vi "Pre Launch Init.vi"(11 "Nested in":refnum<class "test.lvclass">) -> (0 "error out":errorcluster, 3 "Nested out":refnum<class "test.lvclass">)   [LabVIEW 2020, in "test.lvlib" / "test.lvclass"]
doc: "(<B>Filename</B>: Actor Framework.lvlib:Actor.lvclass:Pre Launch Init.vi)\n\nDefines behavior that occurs after the Launch Nested Actor method is invoked but before the actor's Actor Core method begins running.\n\nBy default, this method does nothing. A descendant class may override it to define behavior."
uses:
  test.lvclass
  classes/vna-drivers/liteVNA/VD-settings_status.ctl
  test.lvclass/test.ctl
  <vilib>/ActorFramework/Actor/Actor.lvclass
  classes/vna-drivers/liteVNA/VD-LV-LiteVNA.lvclass
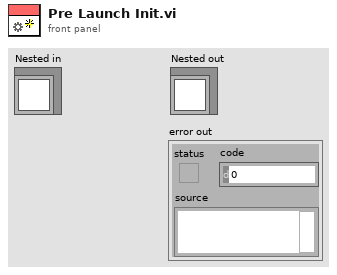
[diagram p1: front panel]
types:
  T1 = typedef "VD-LV-LiteVNA.lvclass/VD-settings_status.ctl" = cluster{"Start [Hz]":u64, "Span [Hz]":u64, "Stop [Mhz]":u64, "Number of points #":u16, "Sample Average #":u16}
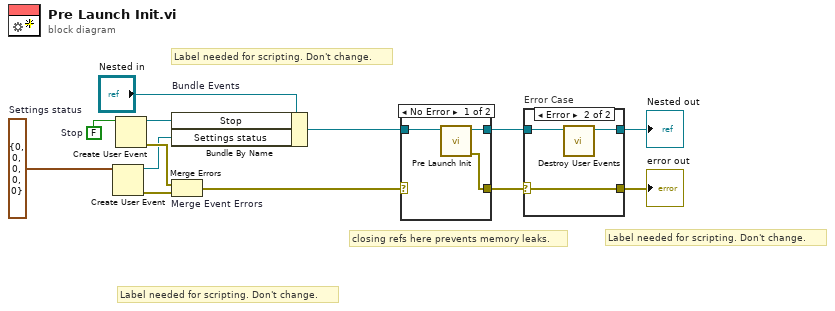
[diagram p0: block diagram]
diagram:
  w3 = T1 {"Start [Hz]"=0, "Span [Hz]"=0, "Stop [Mhz]"=0, "Number of points #"=0, "Sample Average #"=0}  # Settings status
  w12 = FALSE  # Stop
  # "Label needed for scripting. Don't change."
  # "Label needed for scripting. Don't change."
  # "Label needed for scripting. Don't change."
  # "closing refs here prevents memory leaks."
  n1 = Create User Event(user event datatype=w3) -> (user event=w2:refnum<user-event>, error out=w1:errorcluster)  [unwired: 1 in]
  n2 = Create User Event(user event datatype=w12) -> (user event=w9:refnum<user-event>, error out=w11:errorcluster)  [unwired: 1 in]
  n3 = Bundle By Name "Bundle Events"(cluster="Nested in", "Stop"=w9, "Settings status"=w2) -> (w6:refnum<class "test.lvclass">)
  n4 = Merge Errors "Merge Event Errors"(w11, w1) -> (w5:errorcluster)
  n5 = case shown="No Error" w5 {
    selector: w5 -> [_ w18]
    tunnel: [w16 w17] -> w7
    tunnel: w6 -> [w15 w17]
    tunnel: [w14 w18] -> w4
    frame No Error {
      n6 = call-parent "Pre Launch Init.vi"("Actor in"=w15) -> ("error out"=w14:errorcluster, "Actor out"=w16:refnum<class "test.lvclass">)  [unwired: 9 in]
    }
    frame Error {
    }
  }
  n7 = case "Error Case" shown="Error" w4 {
    selector: w4 -> [w19 w23]
    tunnel: w7 -> [w20 w22]
    tunnel: [w20 w21] -> w10
    tunnel: [w19 w23] -> w8
    frame No Error {
    }
    frame Error {
      n8 = call "Destroy User Events.vi"("UI Template in"=w22) -> ("UI Template out"=w21:refnum<class "test.lvclass">)  [unwired: 10 in]
    }
  }
  "error out" <- w8
  "Nested out" <- w10
